vi "simple get func.vi"(10 "task token":refnum<class "null task token.lvclass">, 11 "parameters":variant) -> (1 "error":errorcluster, 2 "data":variant, 3 "data ID":string)   [LabVIEW 2013]
uses:
  task token/null task token.lvclass
  <vilib>/httpClient/ClientHandle.ctl
  <vilib>/LAVA/Variant Repository/Read Variant Repository/Get Read Error.vi
  <userlib>/_OpenG.lib/error/error.llb/Build Error Cluster__ogtk.vi
  <vilib>/LAVA/Variant Repository/Read Variant Repository/Read Variant Repository.xnode
  <vilib>/httpClient/LabVIEWHTTPClient.lvlib
  <userlib>/_OpenG.lib/lvdata/lvdata.llb/Get Data Name__ogtk.vi
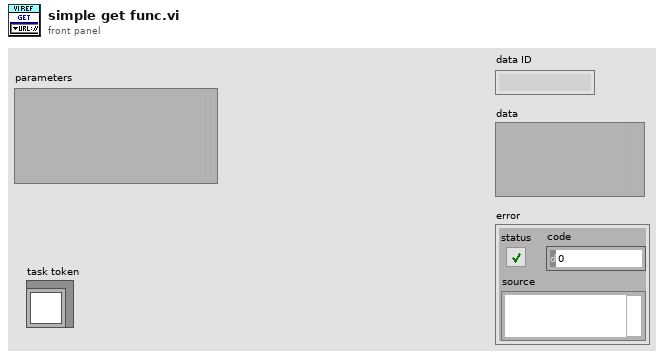
[diagram p1: front panel]
types:
  T1 = typedef "LabVIEWHTTPClient.lvlib/ClientHandle.ctl" = refnum<k1>
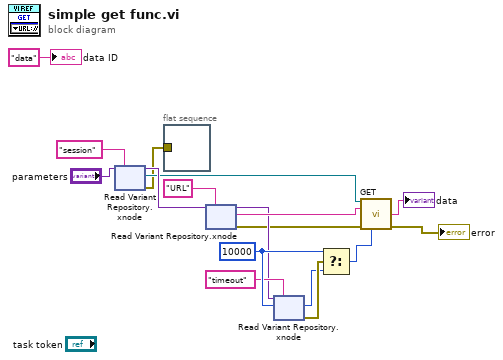
[diagram p0: block diagram]
diagram:
  w8 = 10000 ("timeout (10000)")
  n1 = xnode "Read Variant Repository.xnode"("Variant Repository In"="parameters", "Tag"="session") -> ("Variant Repository Out"=w14:variant, "Value"=w2:T1, "error out"=w1:errorcluster)  [unwired: 2 in]
  n2 = flat-sequence {
    tunnel: w1 -> [_]
    frame #0 {
    }
  }
  n3 = xnode "Read Variant Repository.xnode"("Variant Repository In"=w14, "Tag"="URL") -> ("Variant Repository Out"=w4:variant, "Value"=w15:string, "error out"=w3:errorcluster)  [unwired: 2 in]
  n4 = xnode "Read Variant Repository.xnode"("Variant Repository In"=w4, "Tag"="timeout", "Data Type"=w8) -> ("Value"=w6:i32, "error out"=w9:errorcluster)  [unwired: 1 in, 1 out]
  n5 = Select(t=w8, s=w9, f=w6) -> (s? t:f=w7:i32)
  n6 = call <vilib>:"GET.vi"("client handle"=w2, "url"=w15, "error in (no error)"=w3, "timeout (10000)"=w7) -> ("body"=→"data":string, "error out"=→"error":errorcluster)  [unwired: 8 in, 2 out]
  "data ID" <- "data" ("data ID")
